vi "Bin Photons in Pixels.vi"(6 "# Pixels X":i32, 8 "Error In":errorcluster, 9 "Pixel Duration":u64, 10 "Pixel Start":u64, 11 "Macrotimes":u64[](array[numeric])) -> (0 "Error Out":errorcluster, 1 "Pixel Boundary Indices":i32[](array[numeric]), 3 "Pixel Values":i32[](array[numeric]))   [LabVIEW 2021, in "PTU Files.lvlib"]
uses:
  PTU Files.lvlib
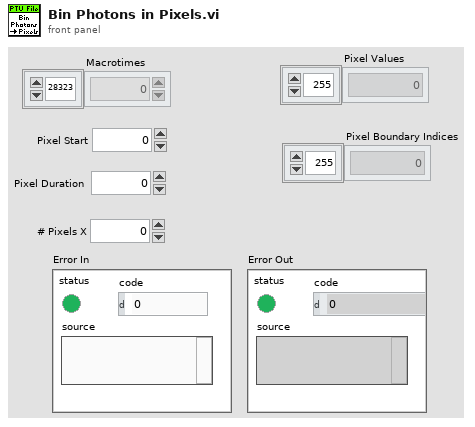
[diagram p1: front panel]
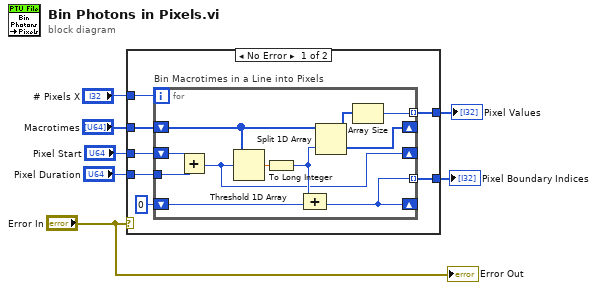
[diagram p0: block diagram]
diagram:
  n1 = case shown="No Error" "Error In" {
    tunnel: "Macrotimes" -> [w14 _]
    tunnel: "Pixel Duration" -> [w13 _]
    tunnel: "# Pixels X" -> [w12 _]
    tunnel: [w11 _] -> w4
    tunnel: [w10 _] -> w2
    tunnel: "Pixel Start" -> [w8 _]
    frame No Error {
      n2 = for "Bin Macrotimes in a Line into Pixels" {
        N: w12 -> [_]
        shift-right: [w23] -> _
        shift-left: w14 -> [w19]
        tunnel: w13 -> [w25]
        tunnel: [w22] -> w11 mode=indexing
        tunnel: [w17] -> w10 mode=indexing
        shift-right: [w17] -> _
        shift-left: 0 -> [w18]
        shift-right: [w15] -> _
        shift-left: w8 -> [w16]
        n3 = Add(x=w16, y=w25) -> (x+y=w15:u64)
        n4 = Threshold 1D Array(2:w15, 3:w19) -> (0:w21:dbl)  [unwired: 1 in]
        n5 = To Long Integer(number=w21) -> (32bit integer=w20:i32)
        n6 = Compound Arithmetic op=ADD(w20, w18) -> (w17:i32)
        n7 = Split 1D Array(array=w19, index=w20) -> (first subarray=w24:u64[], second subarray=w23:u64[])
        n8 = Array Size(array=w24) -> (size(s)=w22:i32)
      }
    }
    frame Error {
    }
  }
  "Pixel Values" <- w4
  "Pixel Boundary Indices" <- w2
  "Error Out" <- "Error In"
